vi "CAN Get CAN Speed Arg.vi"(9 "SpeedBps":u32, 10 "pCanConfig":T1, 11 "DevHandle":i32) -> (2 "pCanConfig out":T1, 3 "function return":i32)   [LabVIEW 2010, in "usb2can.lvlib"]
doc: "int WINAPI CAN_GetCANSpeedArg(int DevHandle,CAN_INIT_CONFIG* pCanConfig, unsigned int SpeedBps);"
uses:
  usb2can.lvlib
  USB2XXX.dll
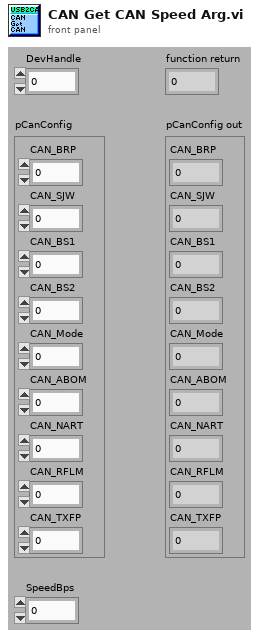
[diagram p1: front panel]
types:
  T1 = cluster{"CAN_BRP":u32, "CAN_SJW":u8, "CAN_BS1":u8, "CAN_BS2":u8, "CAN_Mode":u8, "CAN_ABOM":u8, "CAN_NART":u8, "CAN_RFLM":u8, "CAN_TXFP":u8}
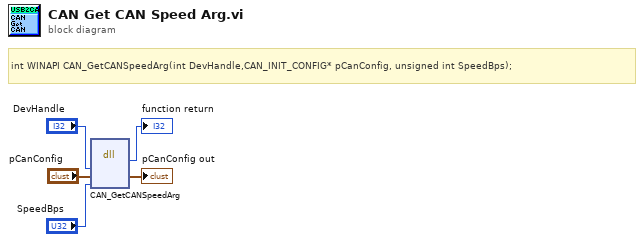
[diagram p0: block diagram]
diagram:
  # "int WINAPI CAN_GetCANSpeedArg(int DevHandle,CAN_INIT_CONFIG* pCanConfig, unsigned int SpeedBps);"
  n1 = dll-call lib="E:/Projects/USB2XXX_Example/sdk/api/Labview/usb2can/USB2XXX.*" fn="CAN_GetCANSpeedArg"("DevHandle"="DevHandle", "pCanConfig"="pCanConfig", "SpeedBps"="SpeedBps") -> (→"function return":i32, "pCanConfig"=→"pCanConfig out":T1)  [unwired: 5 in, 2 out]
